vi "StanfordResSysDG645DelayGeneratorFromDLAY.vi"(11 "ControlArray":refnum<vi>[](array[refnum])) -> ()   [LabVIEW 2021]
uses:
  <vilib>/regexp/Match Regular Expression.xnode
  lib/Hardware/TextControlledInstrum/TextControlledInstrum.lvlib
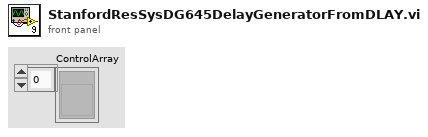
[diagram p1: front panel]
types:
  T1 = cluster{"string array[0]":string, "string array[1]":string}
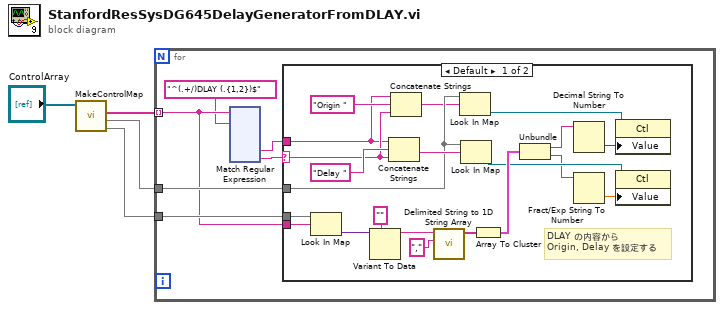
[diagram p0: block diagram]
diagram:
  n1 = call "MakeControlMap.vi"("ControlArray"="ControlArray") -> ("ValueMap out"=w2:map{string, variant}, "ControlMap out"=w1:map{string, refnum<vi>}, "Names"=w3:string[])  [unwired: 7 in, 1 out]
  n2 = for {
    tunnel: w3 -> [w8] mode=indexing
    tunnel: w2 -> [w10]
    tunnel: w1 -> [w9]
    n3 = xnode "Match Regular Expression"("input string"=w8, "regular expression"="^(.+/)DLAY (.{1,2})$") -> ("submatch 1"=w6:string, "submatch 2"=w7:string)  [unwired: 4 in, 5 out]
    n4 = case shown="Default" w7 {
      selector: w7 -> [w149 _]
      tunnel: w10 -> [w145 _]
      tunnel: w9 -> [w147 _]
      tunnel: w8 -> [w144 _]
      tunnel: w6 -> [w131 _]
      frame Default {
        # "DLAY の内容から\nOrigin, Delay を設定する"
        n5 = Look In Map(map=w145, key=w144) -> (value=w143:variant)  [unwired: 1 in, 1 out]
        n6 = Variant To Data(type="", Variant=w143) -> (data=w141:string)  [unwired: 1 in, 1 out]
        n7 = Concatenate Strings(w131, "Delay ", w149) -> (w148:string)
        n8 = Concatenate Strings(w131, "Origin ", w149) -> (w146:string)
        n9 = call <vilib>:"Delimited String to 1D String Array.vi"("delimiter"=",", "delimited string"=w141) -> ("string array"=w139:string[])  [unwired: 9 in]
        n10 = Look In Map(map=w147, key=w146) -> (value=w136:refnum<vi>)  [unwired: 1 in, 1 out]
        n11 = Look In Map(map=w147, key=w148) -> (value=w134:refnum<vi>)  [unwired: 1 in, 1 out]
        n12 = Array To Cluster(array=w139) -> (cluster=w138:T1)
        n13 = Unbundle(w138) -> ("string array[0]"=w137:string, "string array[1]"=w132:string)
        n14 = Decimal String To Number(string=w137) -> (number=w135:i32)  [unwired: 2 in, 1 out]
        n15 = Fract/Exp String To Number(string=w132) -> (number=w133:dbl)  [unwired: 3 in, 1 out]
        n16 = property class="Ctl"(reference=w136, "Value"=w135) -> ()  [unwired: 1 in, 2 out]
        n17 = property class="Ctl"(reference=w134, "Value"=w133) -> ()  [unwired: 1 in, 2 out]
      }
      frame "" {
      }
    }
  }
